vi "Append.vi"(8 "error in (no error)":errorcluster, 10 "SensorData in 2":refnum<class "SensorData.lvclass">, 11 "SensorData in":refnum<class "SensorData.lvclass">) -> (0 "error out":errorcluster, 3 "SensorData out":refnum<class "SensorData.lvclass">)   [LabVIEW 2012, in "Sensor Definition.lvlib" / "SensorData.lvclass"]
uses:
  SensorData.lvclass
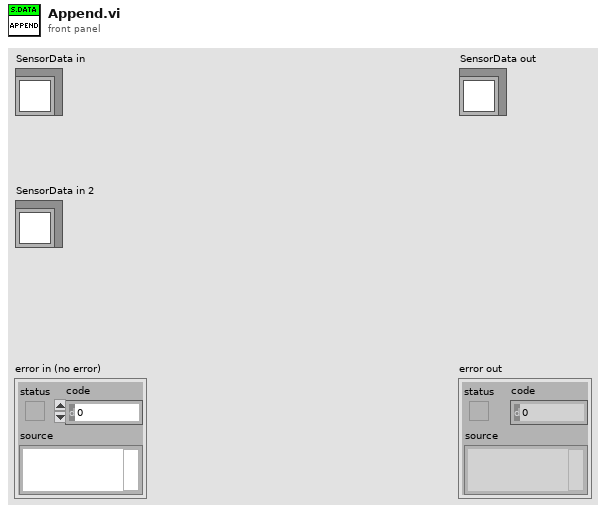
[diagram p1: front panel]
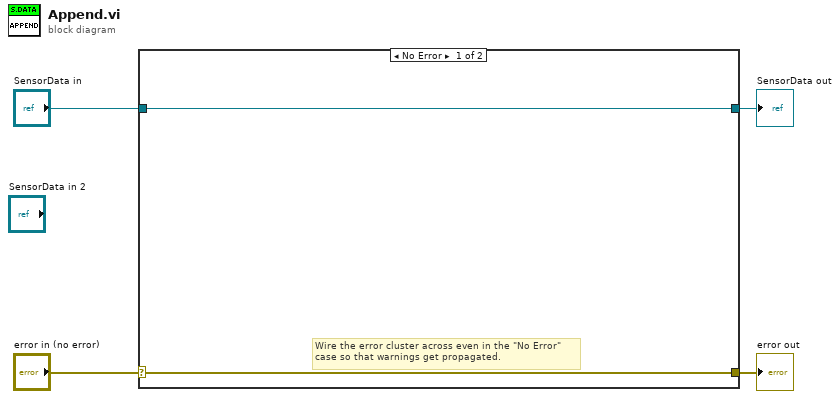
[diagram p0: block diagram]
diagram:
  n1 = case shown="No Error" "error in (no error)" {
    selector: "error in (no error)" -> [w5 w8]
    tunnel: [w5 w8] -> w3
    tunnel: [w6 w7] -> w1
    tunnel: "SensorData in" -> [w6 w7]
    frame No Error {
      # "Wire the error cluster across even in the \"No Error\"\ncase so that warnings get propagated."
    }
    frame Error {
    }
  }
  "error out" <- w3
  "SensorData out" <- w1
